vi "Tree Get Node Wild.vi"(8 "error in (no error)":errorcluster, 10 "Path":string, 11 "Tree DVR in":refnum<data-value>) -> (0 "error out":errorcluster, 2 "Node array out":refnum<data-value>, 3 "Tree DVR out":refnum<data-value>)   [LabVIEW 2012, in "MDSplus.lvlib"]
uses:
  <vilib>/MDSplus/Library/MDSplus.lvlib
  <vilib>/MDSplus/Classes/Tree_Class/Tree.lvclass
  <vilib>/MDSplus/Classes/TreeNodeArray_Class/TreeNodeArray.lvclass
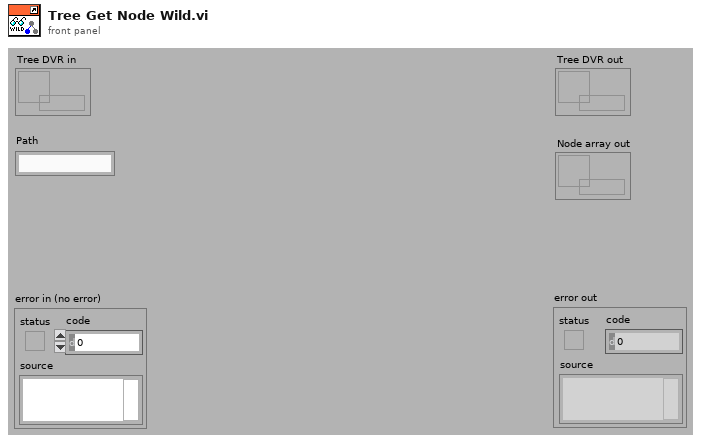
[diagram p1: front panel]
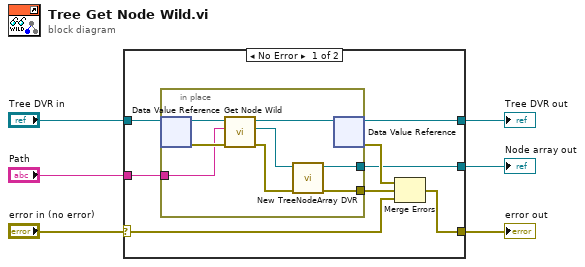
[diagram p0: block diagram]
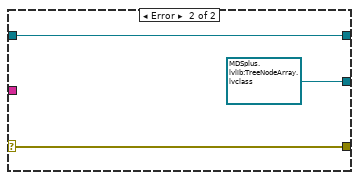
[diagram p2: hidden frame]
diagram:
  n1 = case shown="No Error" "error in (no error)" {
    selector: "error in (no error)" -> [w13 w25]
    tunnel: "Tree DVR in" -> [w14 w24]
    tunnel: [w11 w25] -> w6
    tunnel: [w10 w24] -> w3
    tunnel: [w8 refnum<data-value> refnum ("TreeNode DVR out")] -> w1
    tunnel: "Path" -> [w9 _]
    frame No Error {
      n2 = in-place {
        in-place-border: [w16] -> w7
        in-place-border: w9 -> [w19]
        in-place-border: [w18] -> w8
        n3 = in-place-dvr #1(w14) -> (w22:refnum<class "Tree.lvclass">, w20:errorcluster)
        n4 = call-dynamic "Get Node Wild.vi"("error in (no error)"=w20, "Path"=w19, "Tree in"=w22) -> ("error out"=w17:errorcluster, "Node array out"=w15:refnum<class "TreeNodeArray.lvclass">, "Tree out"=w21:refnum<class "Tree.lvclass">)  [unwired: 6 in]
        n5 = call <vilib>:"New TreeNodeArray DVR.vi"("error in (no error)"=w17, "TreeNodeArray in"=w15) -> ("error out"=w16:errorcluster, "TreeNodeArray DVR out"=w18:refnum<data-value>)  [unwired: 8 in]
        n6 = in-place-dvr #1(w21) -> (w10:refnum<data-value>, w12:errorcluster)
      }
      n7 = Merge Errors(w12, w7, w13) -> (w11:errorcluster)
    }
    frame Error {
    }
  }
  "error out" <- w6
  "Tree DVR out" <- w3
  "Node array out" <- w1
